vi "CopyAssetFiles.vi"(8 "error in (no error)":errorcluster, 11 "VeriStandTestCase in":refnum<class "VeriStandTestCase.lvclass">) -> (0 "error out":errorcluster, 3 "VeriStandTestCase out":refnum<class "VeriStandTestCase.lvclass">)   [LabVIEW 2020, in "VeriStandTestCase.lvclass"]
uses:
  VeriStandTestCase.lvclass
  <vilib>/Utility/error.llb/Trim Whitespace One-Sided.vi
  <userlib>/_OpenG.lib/file/file.llb/File Exists - Scalar__ogtk.vi
  <userlib>/_OpenG.lib/file/file.llb/openg_file.lvlib
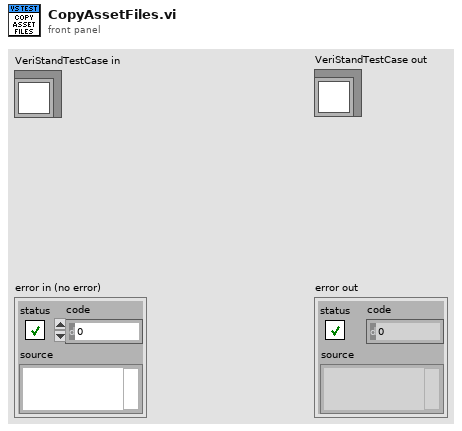
[diagram p1: front panel]
types:
  T1 = typedef "VeriStandTestUtilities.lvlib/GatewayConfiguration.ctl" = cluster{"Enable Remote Gateway":bool, "GatewayIP":string, "Username":string, "System Path":string}
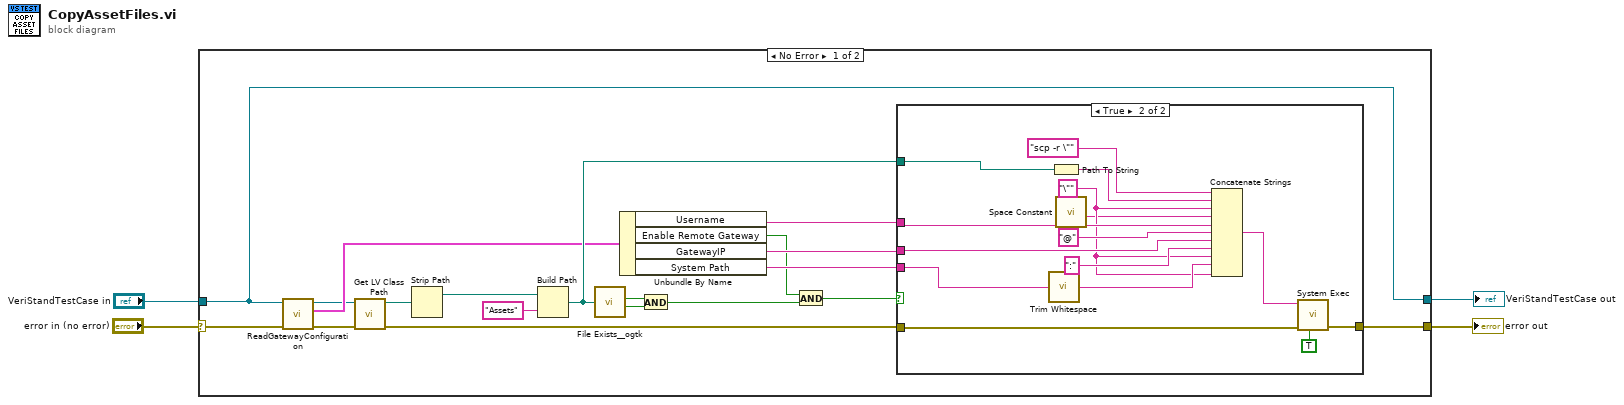
[diagram p0: block diagram]
diagram:
  n1 = case shown="No Error" "error in (no error)" {
    selector: "error in (no error)" -> [w23 w41]
    tunnel: [w5 w41] -> w3
    tunnel: [w7 w40] -> w1
    tunnel: "VeriStandTestCase in" -> [w7 w40]
    frame No Error {
      n2 = call "ReadGatewayConfiguration.vi"("error in (no error)"=w23, "VeriStandTestCase in"=w7) -> ("error out"=w19:errorcluster, "Gateway Configuration"=w10:T1, "VeriStandTestCase out"=w8:refnum<class "VeriStandTestCase.lvclass">)  [unwired: 7 in]
      n3 = call <vilib>:"Get LV Class Path.vi"("error in (no error)"=w19, "object"=w8) -> ("error out"=w6:errorcluster, "class path"=w22:path)  [unwired: 8 in]
      n4 = Strip Path(path=w22) -> (stripped path=w11:path)  [unwired: 1 out]
      n5 = Build Path(base path=w11, name or relative path="Assets") -> (appended path=w17:path)
      n6 = call-poly <userlib>:"File Exists__ogtk.vi"("file path"=w17) -> ("is directory"=w15:bool, "exists"=w20:bool)  [unwired: 6 in]
      n7 = Unbundle By Name(w10) -> ("Username"=w16:string, "Enable Remote Gateway"=w9:bool, "GatewayIP"=w14:string, "System Path"=w12:string)
      n8 = And(x=w15, y=w20) -> (x .and. y?=w13:bool)
      n9 = And(x=w9, y=w13) -> (x .and. y?=w18:bool)
      n10 = case shown="True" w18 {
        tunnel: w17 -> [_ w39]
        tunnel: w16 -> [_ w33]
        tunnel: w14 -> [_ w35]
        tunnel: w12 -> [_ w30]
        tunnel: w6 -> [w24 w28]
        tunnel: [w24 w26] -> w5
        frame False {
        }
        frame True {
          w31 = "\"" ("string")
          n11 = call <vilib>:"Trim Whitespace.vi"("string"=w30) -> ("trimmed string"=w32:string)  [unwired: 1 in]
          n12 = Path To String(path=w39) -> (string=w37:string)
          n13 = call <vilib>:"Space Constant.vi"() -> ("String"=w29:string)
          n14 = Concatenate Strings("scp -r \"" ("command line"), w37, w31, w29, w33, "@" ("string"), w35, ":" ("string"), w31, w32, w31) -> (w27:string)
          n15 = call <vilib>:"System Exec.vi"("run minimized? (F)"=TRUE, "error in (no error)"=w28, "command line"=w27) -> ("error out"=w26:errorcluster)  [unwired: 5 in, 3 out]
        }
      }
    }
    frame Error {
    }
  }
  "error out" <- w3
  "VeriStandTestCase out" <- w1
